vi "Main_Transfer.vi"() -> ()   [LabVIEW 2020]
uses:
  <vilib>/vision/NI_Vision_Development_Module.lvlib
panel:
  in  "h":i32=10 min=1 max=5000 step=1
  in  "w":i32=1 min=1 max=5000 step=1
  out "Elaps ms":u32
  in  "Send Image":bool
  out "Path to Python script":path
  in  "Stop":bool
  out "Answer":string
  in  "Ping":bool
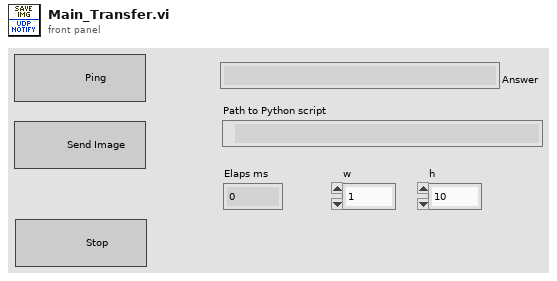
[diagram p1: front panel]
types:
  T1 = enum8{"Enabled", "Disabled", "Disabled and Grayed Out"}
  T2 = typedef "Image Type" = u32
  T3 = cluster{"Rows Per Strip":i32, "Photometric":i32, "Compression Type":i32}
  T4 = typedef "IMAQ Image.ctl" = refnum<image>
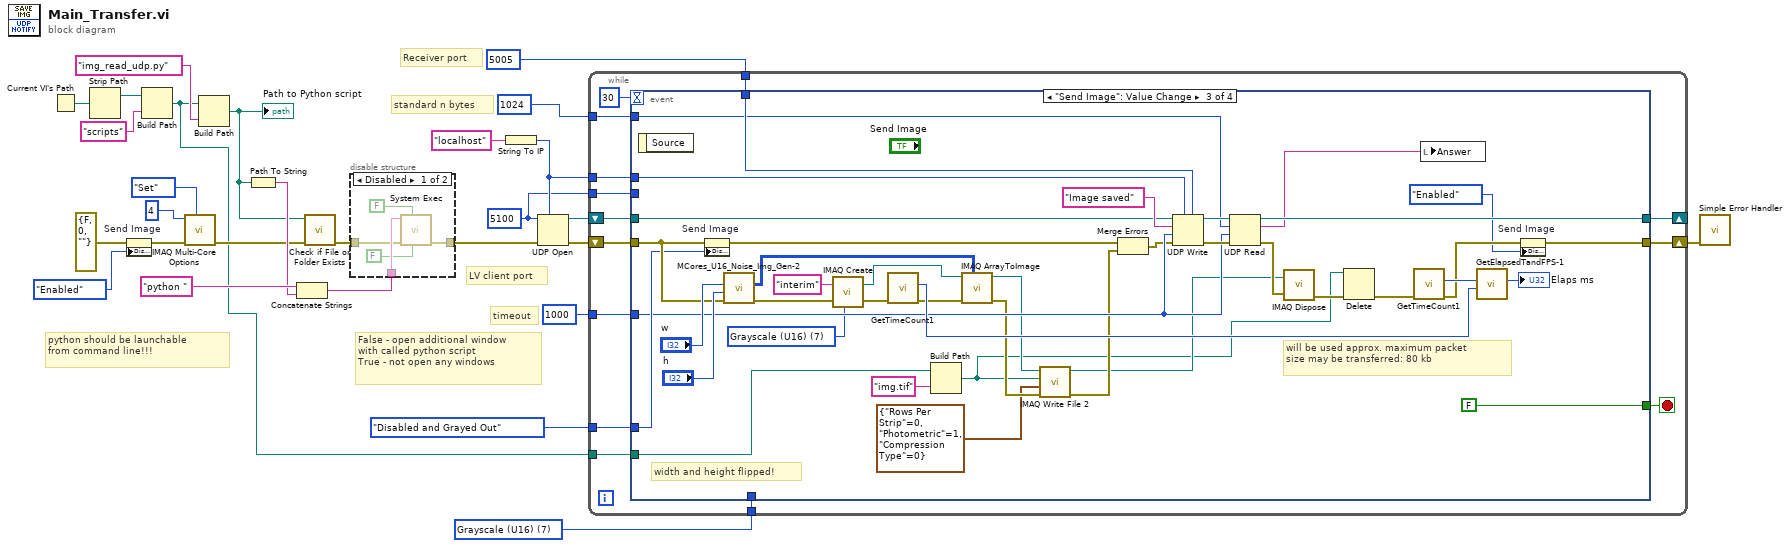
[diagram p0: block diagram]
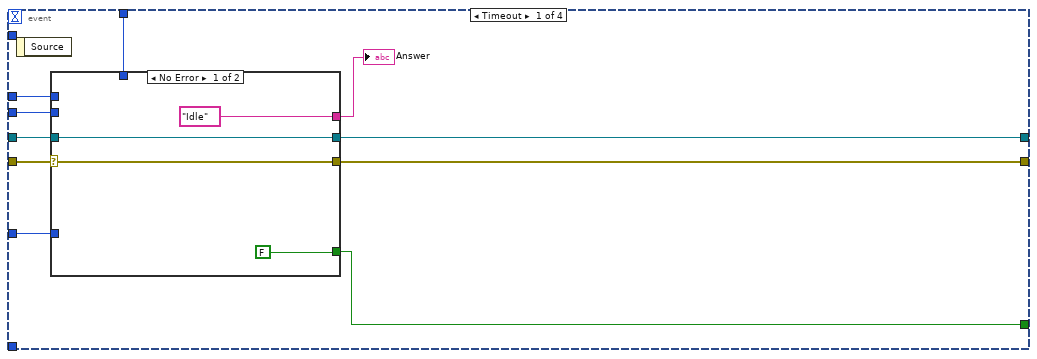
[diagram p3: hidden frame]
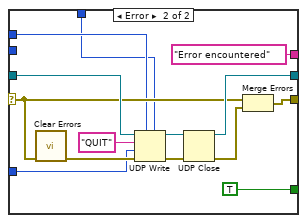
[diagram p4: hidden frame]
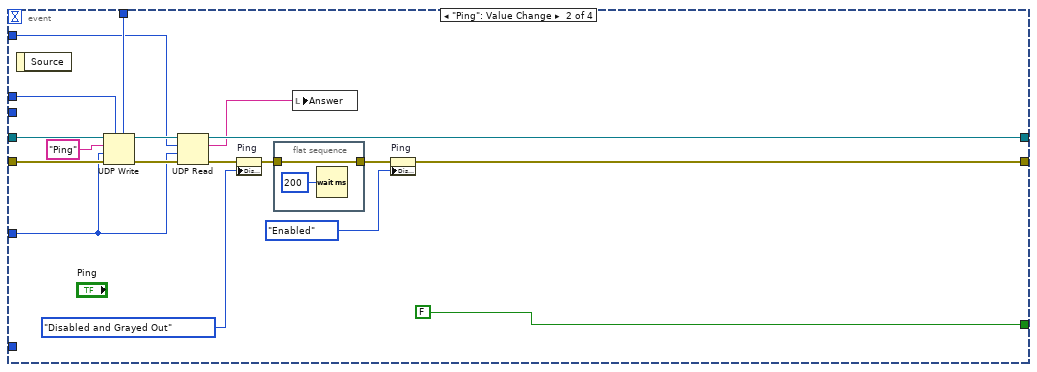
[diagram p5: hidden frame]
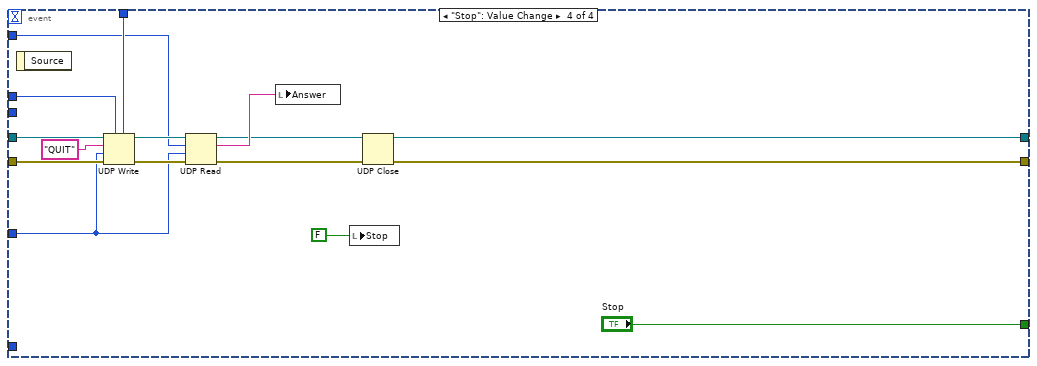
[diagram p6: hidden frame]
diagram:
  w12 = T2 7 items=["Grayscale (U8)", "Grayscale (I16)", "Grayscale (SGL)", "Complex (CSG)", "RGB (U32)", "HSL (U32)", "RGB (U64)", "Grayscale (U16)"] ("Image Type")
  w15 = u16 5100 ("remote port or service name")
  # "standard n bytes"
  # "timeout"
  # "Receiver port"
  # "LV client port"
  # "False - open additional window\nwith called python script\nTrue - not open any windows"
  # "python should be launchable \nfrom command line!!!"
  n1 = Current VI's Path() -> (path=w27:path)
  n2 = Strip Path(path=w27) -> (stripped path=w2:path)  [unwired: 1 out]
  n3 = property on="Send Image" class="Bool"(error in=errorcluster {"status"=FALSE, "code"=0, "source"=""} ("error in (no error)"), "DisabledEnum"=T1."Enabled" ("Disabled")) -> (error out=w6:errorcluster)  [unwired: 1 in, 1 out]
  n4 = Build Path(base path=w2, name or relative path="scripts" ("string")) -> (appended path=w1:path)
  n5 = call "IMAQ Multi-Core Options"("Get/Set Number of Cores (Get)"=enum32{"Get", "Set", "Set Max Available"}."Set", "error in (no error)"=w6, "Specified Number of Cores"=u32 4) -> ("error out"=w3:errorcluster)  [unwired: 7 in, 1 out]
  n6 = Build Path(base path=w1, name or relative path="img_read_udp.py" ("string")) -> (appended path=w22:path)
  "Path to Python script" <- w22
  n7 = Path To String(path=w22) -> (string=w23:string)
  n8 = Concatenate Strings("python " ("command line"), w23) -> (w25:string)
  n9 = call <vilib>:"Check if File or Folder Exists.vi"("error in (no error)"=w3, "path"=w22) -> ("error out"=w21:errorcluster)  [unwired: 7 in, 2 out]
  n10 = disable-structure shown="Disabled" {
    disable-tunnel: w25 -> [w33 _]
    disable-tunnel: [w32 w34] -> w20
    disable-tunnel: w21 -> [w30 w34]
    frame Disabled {
      n11 = call <vilib>:"System Exec.vi"("run minimized? (F)"=FALSE, "wait until completion? (T)"=FALSE, "error in (no error)"=w30, "command line"=w33) -> ("error out"=w32:errorcluster)  [unwired: 4 in, 3 out]
    }
    frame Enabled {
    }
  }
  n12 = String To IP(1:"localhost" ("address")) -> (0:w16:u32)
  n13 = UDP Open(7:w16, 8:w20, 11:w15) -> (port=w18:refnum<k16>, 0:w19:errorcluster)  [unwired: 2 in, 1 out]
  n14 = while {
    shift-right: [w45] -> _
    shift-left: w18 -> [w46]
    shift-right: [w43] -> w28
    shift-left: w19 -> [w47]
    tunnel: w16 -> [w41]
    tunnel: w15 -> [w42]
    tunnel: u16 5005 ("remote port or service name") -> [w40]
    tunnel: 1000 -> [w39]
    tunnel: w12 -> [w38]
    tunnel: T1."Disabled and Grayed Out" ("Disabled") -> [w37]
    tunnel: 1024 ("bytes to read") -> [w36]
    tunnel: w1 -> [w35]
    stop <- w44 stop-if-true
    n15 = event shown="[2] \"Send Image\": Value Change" {
      selector: _ -> [_ _ _ _]
      dyn-events: _ -> [_ _ _ _]
      timeout: 30 -> [_ _ _ _]
      tunnel: [w54 FALSE ("Stop") FALSE ("Stop") "Stop"] -> w44
      tunnel: w47 -> [w58 w88 w125 w148]
      tunnel: w46 -> [w57 w87 w136 w149]
      tunnel: [w56 w83 w134 w150] -> w45
      tunnel: [w55 w90 w122 w151] -> w43
      tunnel: w42 -> [w52 _ _ _]
      tunnel: w41 -> [w51 w80 w129 w141]
      tunnel: w40 -> [w50 w79 w128 w140]
      tunnel: w39 -> [w49 w78 w118 w138]
      tunnel: w38 -> [_ _ _ _]
      tunnel: w37 -> [_ _ w124 _]
      tunnel: w36 -> [_ w77 w117 w139]
      tunnel: w35 -> [_ _ w103 _]
      event Timeout {
        n16 = event-data() -> ()  [unwired: 1 in, 1 out]
        n17 = case shown="No Error" w58 {
          selector: w58 -> [w61 w67]
          tunnel: [w62 w74] -> w56
          tunnel: w57 -> [w62 w73]
          tunnel: [w61 w68] -> w55
          tunnel: [FALSE ("Stop") TRUE ("Stop")] -> w54
          tunnel: ["Idle" ("Answer") "Error encountered" ("Answer")] -> w53
          tunnel: w52 -> [_ _]
          tunnel: w51 -> [_ w65]
          tunnel: w50 -> [_ w64]
          tunnel: w49 -> [_ w63]
          frame No Error {
          }
          frame Error {
            n18 = call <vilib>:"Clear Errors.vi"("error in (no error)"=w67) -> ("error out"=w72:errorcluster)  [unwired: 5 in, 1 out]
            n19 = UDP Write(address=w65, port or service name=w64, connection ID=w73, data in="QUIT", 8:w72, 9:w63) -> (error out=w71:errorcluster, 3:w69:refnum<k16>)
            n20 = UDP Close(connection ID=w69, 8:w71) -> (connection ID out=w74:refnum<k16>, error out=w66:errorcluster)
            n21 = Merge Errors(w67, w66) -> (w68:errorcluster)
          }
        }
        "Answer" <- w53
      }
      event "Ping": Value Change {
        n22 = event-data() -> ()  [unwired: 1 in, 1 out]
        n23 = UDP Write(address=w80, port or service name=w79, connection ID=w87, data in="Ping", 8:w88, 9:w78) -> (error out=w85:errorcluster, 3:w84:refnum<k16>)
        n24 = UDP Read(connection ID=w84, max size (548)=w77, timeout ms (25000)=w78, 8:w85) -> (data out=w81:string, error out=w82:errorcluster, 3:w83:refnum<k16>)  [unwired: 2 out]
        n25 = property on="Ping" class="Bool"(error in=w82, "DisabledEnum"=T1."Disabled and Grayed Out" ("Disabled")) -> (error out=w93:errorcluster)  [unwired: 1 in, 1 out]
        n26 = flat-sequence {
          tunnel: w93 -> [w95]
          tunnel: [w95] -> w91
          frame #0 {
            n27 = Wait (ms)(milliseconds to wait=u32 200) -> ()  [unwired: 1 out]
          }
        }
        n28 = local write "Answer"(w81) -> ()
        n29 = property on="Ping" class="Bool"(error in=w91, "DisabledEnum"=T1."Enabled" ("Disabled")) -> (error out=w90:errorcluster)  [unwired: 1 in, 1 out]
      }
      event "Send Image": Value Change {
        w114 = T2 7 items=["Grayscale (U8)", "Grayscale (I16)", "Grayscale (SGL)", "Complex (CSG)", "RGB (U32)", "HSL (U32)", "RGB (U64)", "Grayscale (U16)"] ("Image Type")
        # "width and height flipped!"
        # "will be used approx. maximum packet \nsize may be transferred: 80 kb"
        n30 = event-data() -> ()  [unwired: 1 in, 1 out]
        n31 = property on="Send Image" class="Bool"(error in=w125, "DisabledEnum"=w124) -> (error out=w116:errorcluster)  [unwired: 1 in, 1 out]
        n32 = call "MCores_U16_Noise_Img_Gen-2.vi"("error IN"=w125, "[IN] Width"="h", "[IN] Height"="w") -> ("error OUT"=w112:errorcluster, "[OUT] U16 Pixel Img"=w108:u16[][])  [unwired: 7 in]
        n33 = call "IMAQ Create"("Image Name"="interim", "Image Type"=w114, "error in (no error)"=w112) -> ("New Image"=w109:T4, "error out"=w111:errorcluster)  [unwired: 2 in]
        n34 = call "GetTimeCount1.vi"("error IN"=w111) -> ("error OUT"=w110:errorcluster, "[OUT] Timer Count"=w131:u32)  [unwired: 9 in]
        n35 = Build Path(base path=w103, name or relative path="img.tif" ("string")) -> (appended path=w97:path)
        n36 = call "IMAQ ArrayToImage"("Image Pixels (U16)"=w108, "error in (no error)"=w110, "Image"=w109) -> ("error out"=w107:errorcluster, "Image Out"=w106:T4)  [unwired: 7 in]
        n37 = call-poly "IMAQ Write File 2"("error in (no error)"=w107, "TIFF Options"=T3 {"Rows Per Strip"=0, "Photometric"=1, "Compression Type"=0}, "File Path"=w97, "Image"=w106) -> ("error out"=w105:errorcluster, "Image Out (duplicate)"=w100:T4)  [unwired: 6 in]
        n38 = Merge Errors(w116, w105) -> (w115:errorcluster)
        n39 = UDP Write(address=w129, port or service name=w128, connection ID=w136, data in="Image saved", 8:w115, 9:w118) -> (error out=w119:errorcluster, 3:w120:refnum<k16>)
        n40 = UDP Read(connection ID=w120, max size (548)=w117, timeout ms (25000)=w118, 8:w119) -> (data out=w133:string, error out=w101:errorcluster, 3:w134:refnum<k16>)  [unwired: 2 out]
        n41 = call "IMAQ Dispose"("Image"=w100, "error in (no error)"=w101) -> ("error out"=w99:errorcluster)  [unwired: 4 in]
        n42 = Delete(path (use dialog)=w97, error in=w99) -> (error out=w98:errorcluster)  [unwired: 3 in, 2 out]
        n43 = call "GetTimeCount1.vi"("error IN"=w98) -> ("error OUT"=w123:errorcluster, "[OUT] Timer Count"=w132:u32)  [unwired: 9 in]
        n44 = local write "Answer"(w133) -> ()
        n45 = call "GetElapsedTandFPS-1.vi"("[IN] Timer Count Before ALL [ms]"=w131, "[IN] Timer Count After ALL [ms]"=w132) -> ("[OUT] Elapsed time [ms]"=→"Elaps ms":u32)  [unwired: 3 in, 2 out]
        n46 = property on="Send Image" class="Bool"(error in=w123, "DisabledEnum"=T1."Enabled" ("Disabled")) -> (error out=w122:errorcluster)  [unwired: 1 in, 1 out]
      }
      event "Stop": Value Change {
        n47 = event-data() -> ()  [unwired: 1 in, 1 out]
        n48 = UDP Write(address=w141, port or service name=w140, connection ID=w149, data in="QUIT", 8:w148, 9:w138) -> (error out=w145:errorcluster, 3:w146:refnum<k16>)
        n49 = UDP Read(connection ID=w146, max size (548)=w139, timeout ms (25000)=w138, 8:w145) -> (data out=w143:string, error out=w144:errorcluster, 3:w142:refnum<k16>)  [unwired: 2 out]
        n50 = local write "Answer"(w143) -> ()
        n51 = local write "Stop"(FALSE ("Stop")) -> ()
        n52 = UDP Close(connection ID=w142, 8:w144) -> (connection ID out=w150:refnum<k16>, error out=w151:errorcluster)
      }
    }
  }
  n53 = call <vilib>:"Simple Error Handler.vi"("error in (no error)"=w28) -> ()  [unwired: 4 in, 5 out]
